vi "U8ArrayToU32Array.vi"(1 "U8-bit Array":u8[](array[numeric])) -> (0 "U32-bit Array":u32[](array[numeric]))   [LabVIEW 2011]
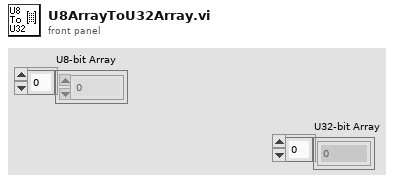
[diagram p1: front panel]
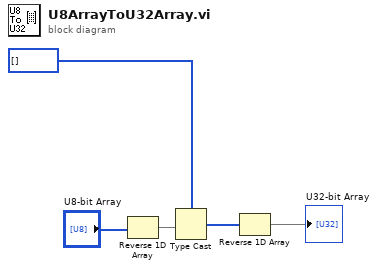
[diagram p0: block diagram]
diagram:
  n1 = Reverse 1D Array(array="U8-bit Array") -> (reversed array=w4:u8[])
  n2 = Type Cast(type=u32[] [], x=w4) -> (*(type *) &x=w2:u32[])
  n3 = Reverse 1D Array(array=w2) -> (reversed array=→"U32-bit Array":u32[])
